vi "Set Package Paths.vi"(4 "ms timeout (-1)":i32=-1, 8 "error in":errorcluster, 9 "Cpaths":string[](array[string]), 10 "Lpaths":string[](array[string]), 11 "GLue in":refnum<class "class.GLue.lvclass">) -> (0 "error out":errorcluster, 3 "GLue out":refnum<class "class.GLue.lvclass">)   [LabVIEW 2014, in "GLue.lvlib"]
doc: "Set the paths to search for Lua and C modules, see http://www.lua.org/manual/5.2/manual.html#pdf-package.searchpath for further details.\n\n<B>Parameter(s) </B>\n-----------------\n\n- <B>GLue in:</B> Reference to the GLue instance.\n\n- <B>Lpaths:</B> An array of possible paths to Lua script modules.\n\n- <B>Cpaths:</B> An array of possible paths to compiled C modules.\n\n- <B>ms timeout (-1):</B> The time to wait for the GLue reference to become available. A value of '-1' specifies an infinite timeout.\n\n- <B>error in:</B> Describes error conditions that occur before this VI runs. This input provides standard error in functionality. \n\n- <B>GLue out:</B> Reference to the GLue instance.\n\n- <B>error out:</B> Contains error information. This output provides standard error out functionality."
uses:
  GLue.lvlib
  Private/Class/class.GLue.lvclass
panel:
  # "Input"
  # "Output"
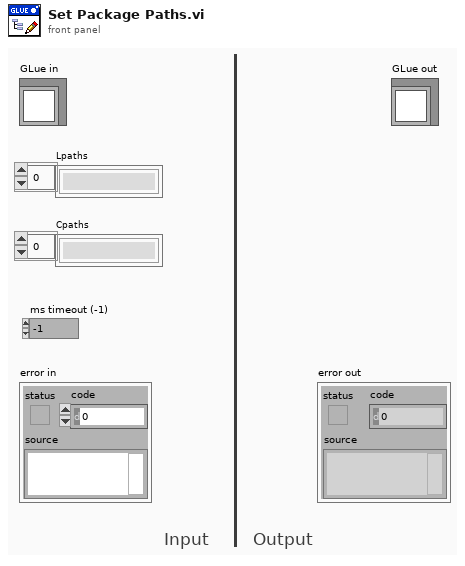
[diagram p1: front panel]
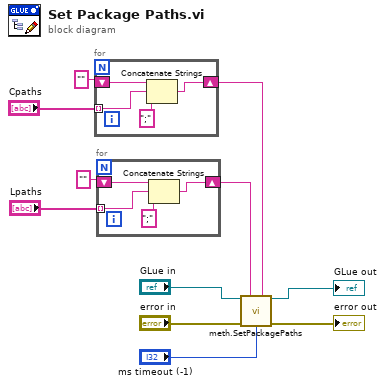
[diagram p0: block diagram]
diagram:
  n1 = for {
    tunnel: "Cpaths" -> [w14] mode=indexing
    shift-right: [w12] -> w4
    shift-left: "" ("delimiter (Tab)") -> [w15]
    n2 = Concatenate Strings(w15, w14, ";" ("string")) -> (w12:string)
  }
  n3 = for {
    tunnel: "Lpaths" -> [w18] mode=indexing
    shift-right: [w16] -> w1
    shift-left: "" ("delimiter (Tab)") -> [w19]
    n4 = Concatenate Strings(w19, w18, ";" ("string")) -> (w16:string)
  }
  n5 = call "meth.SetPackagePaths.vi"("class.GLue in"="GLue in", "Lpaths"=w1, "Cpaths"=w4, "error in"="error in", "ms timeout (-1)"="ms timeout (-1)") -> ("class.GLue out"=→"GLue out":refnum<class "class.GLue.lvclass">, "error out"=→"error out":errorcluster)  [unwired: 9 in]
